vi "Matlab_CloseAllFigures.vi"(8 "Error In":errorcluster) -> (0 "Error Out":errorcluster)   [LabVIEW 2014]
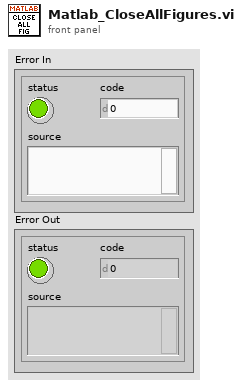
[diagram p1: front panel]
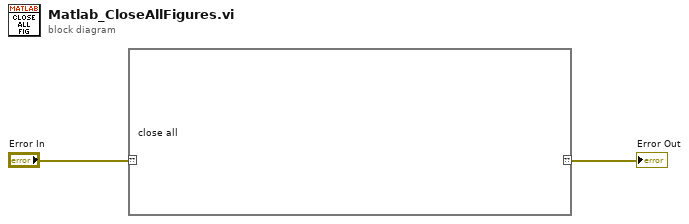
[diagram p0: block diagram]
diagram:
  n1 = script code="close all"("??"="Error In") -> ("??"=→"Error Out":errorcluster)
